vi "AAP_Control_Test.vi"() -> ()   [LabVIEW 2019]
uses:
  <vilib>/Powertrain Controls/Device Drivers/Engine Position Tracking/EPTx/RevA/RT/EPTx - RevA - RT.lvlib
  <vilib>/Powertrain Controls/Device Drivers/Engine Position Tracking/EPTx/RevA/FPGA/Controls/EPTxAAPControl.ctl
  <vilib>/Powertrain Controls/Device Drivers/Engine Position Tracking/EPTx/RevA/FPGA/EPTx - RevA - FPGA.lvlib
  <vilib>/Powertrain Controls/Device Drivers/Engine Position Tracking/EPTx/RevA/RT/Controls/EPTxAAPControl.ctl
panel:
  in  "Cylinder TDC [Absolute CAD]":sgl
  in  "EPTxAAPControl 2":T1
  out "EPTxAAPControl":T2
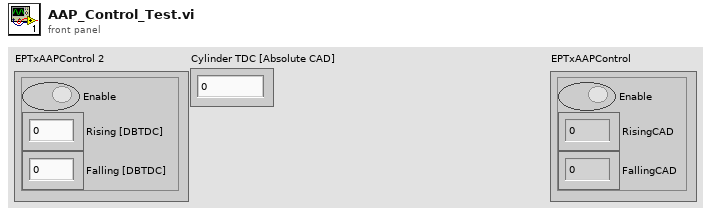
[diagram p1: front panel]
types:
  T1 = typedef "EPTx - RevA - RT.lvlib/EPTxAAPControl.ctl" = cluster{"Enable":bool, "Rising [DBTDC]":sgl, "Falling [DBTDC]":sgl}
  T2 = typedef "EPTx - RevA - FPGA.lvlib/EPTxAAPControl.ctl" = cluster{"Enable":bool, "RisingCAD":fxp<+,18,11>, "FallingCAD":fxp<+,18,11>}
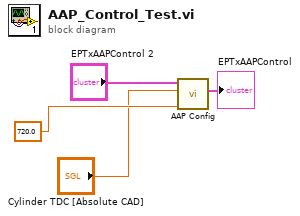
[diagram p0: block diagram]
diagram:
  n1 = call <vilib>:"AAP Config.vi"("Max CAD"=sgl 720.0 ("Cylinder TDC [Absolute CAD]"), "Cylinder TDC [Absolute CAD]"="Cylinder TDC [Absolute CAD]", "EPTxAAPControl"="EPTxAAPControl 2") -> ("EPTxAAPControl"=→"EPTxAAPControl":T2)  [unwired: 8 in]
